vi "sensor_messung.vi"(8 "error in (no error)":errorcluster, 10 "Sensorkoord [P1 P2]":dbl[][](array[numeric]), 11 "Kreisquadrant in":refnum<class "Kreisquadrant.lvclass">) -> (0 "error out":errorcluster, 1 "Sensor auf Linie":bool, 2 "Schnittpunkt":dbl[](array[numeric]), 3 "Kreisquadrant out":refnum<class "Kreisquadrant.lvclass">)   [LabVIEW 2019, in "Kreisquadrant.lvclass"]
uses:
  Kreisquadrant.lvclass
  Kreisquadrant.lvclass/Kreisquadrant.ctl
  <vilib>/Analysis/baseanly.llb/Real Dot Product.vi
  <vilib>/Analysis/NI_AALPro.lvlib
  <vilib>/Analysis/NI_AALBase.lvlib
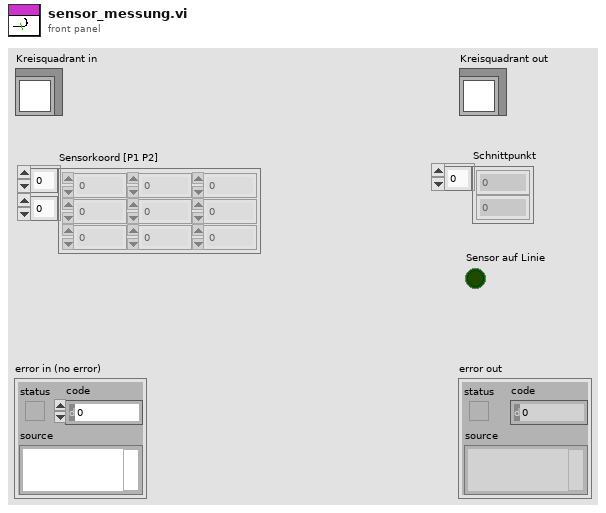
[diagram p1: front panel]
types:
  T1 = typedef "Quadrant.ctl" = enum16{"oben_rechts", "oben_links", "unten_links", "unten_rechts"}
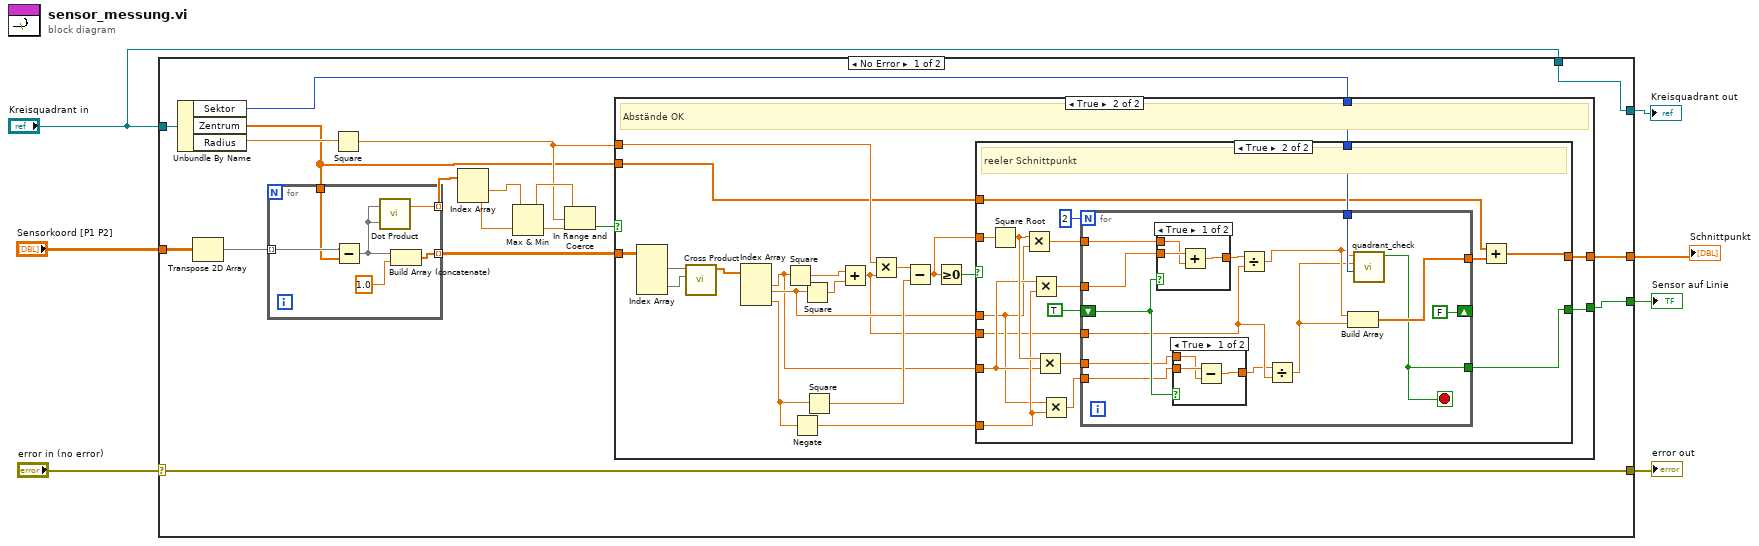
[diagram p0: block diagram]
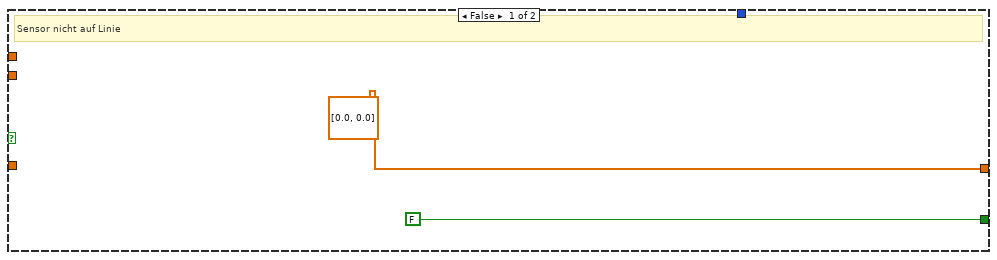
[diagram p2: hidden frame]
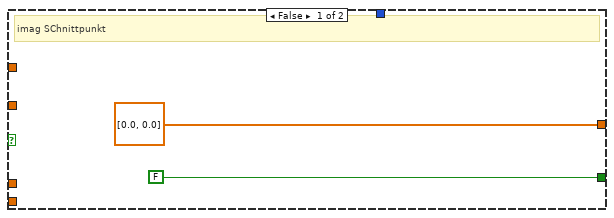
[diagram p3: hidden frame]
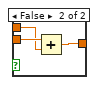
[diagram p4: hidden frame]
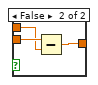
[diagram p5: hidden frame]
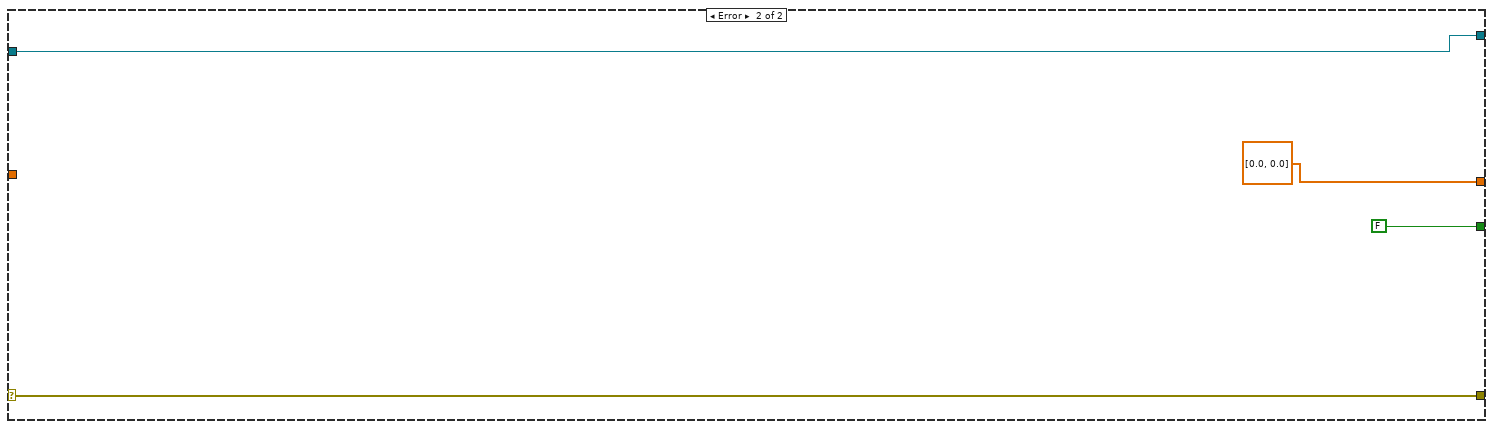
[diagram p6: hidden frame]
diagram:
  n1 = case shown="No Error" "error in (no error)" {
    selector: "error in (no error)" -> [w25 w102]
    tunnel: [w25 w102] -> w6
    tunnel: "Kreisquadrant in" -> [w24 w99]
    tunnel: "Sensorkoord [P1 P2]" -> [w23 _]
    tunnel: [w12 dbl[] [0.0, 0.0]] -> w4
    tunnel: [w13 FALSE ("Quadrant OK")] -> w3
    tunnel: [w9 w99] -> w2
    tunnel: "Kreisquadrant in" -> [w9 _]
    frame No Error {
      n2 = Unbundle By Name(w24) -> ("Sektor"=w10:T1, "Zentrum"=w8:dbl[], "Radius"=w20:dbl)
      n3 = Transpose 2D Array(2D array=w23) -> (transposed array=w22:dbl[][])
      n4 = for {
        tunnel: w22 -> [w98] mode=indexing
        tunnel: w8 -> [w97]
        tunnel: [w96] -> w21 mode=indexing
        tunnel: [w93] -> w19 mode=indexing
        n5 = Subtract(x=w98, y=w97) -> (x-y=w94:dbl[])
        n6 = call-poly <vilib>:"Dot Product.vi"("Y Vector"=w94, "X Vector"=w94) -> ("X * Y"=w93:dbl)  [unwired: 1 out]
        n7 = Build Array (concatenate)(w94, 1.0) -> (w96:dbl[])
      }
      n8 = Square(x=w20) -> (x^2=w11:dbl)
      n9 = Index Array(array=w19) -> (element #1=w18:dbl, element #2=w17:dbl)  [unwired: 2 in]
      n10 = Max & Min(x=w18, y=w17) -> (max(x,y)=w16:dbl, min(x,y)=w15:dbl)
      n11 = In Range and Coerce(upper limit=w16, x=w11, lower limit=w15) -> (In Range?=w14:bool)  [unwired: 1 out]
      n12 = case shown="True" w14 {
        tunnel: w21 -> [_ w47]
        tunnel: [FALSE w36] -> w13
        tunnel: [dbl[] [0.0, 0.0] w37] -> w12
        tunnel: w11 -> [_ w41]
        tunnel: w10 -> [_ w30]
        tunnel: w8 -> [_ w29]
        frame False {
          # "Sensor nicht auf Linie"
        }
        frame True {
          # "Abstände OK"
          n13 = Index Array(array=w47) -> (element #1=w46:dbl[], element #2=w45:dbl[])  [unwired: 4 in]
          n14 = call <vilib>:"Cross Product.vi"("B Vector"=w45, "A Vector"=w46) -> ("Cross Product"=w44:dbl[])  [unwired: 8 in, 1 out]
          n15 = Index Array(array=w44) -> (element #1=w33:dbl, element #2=w34:dbl, element #3=w32:dbl)  [unwired: 3 in]
          n16 = Square(x=w33) -> (x^2=w42:dbl)
          n17 = Negate(x=w32) -> (-x=w28:dbl)
          n18 = Square(x=w34) -> (x^2=w43:dbl)
          n19 = Square(x=w32) -> (x^2=w39:dbl)
          n20 = Add(x=w42, y=w43) -> (x+y=w31:dbl)
          n21 = Multiply(x=w41, y=w31) -> (x*y=w40:dbl)
          n22 = Subtract(x=w40, y=w39) -> (x-y=w35:dbl)
          n23 = Greater Or Equal To 0?(x=w35) -> (x >= 0?=w38:bool)
          n24 = case shown="True" w38 {
            tunnel: [dbl[] [0.0, 0.0] w50] -> w37
            tunnel: [FALSE w52] -> w36
            tunnel: w35 -> [_ w66]
            tunnel: w34 -> [_ w62]
            tunnel: w33 -> [_ w63]
            tunnel: w28 -> [_ w64]
            tunnel: w31 -> [_ w57]
            tunnel: w30 -> [_ w54]
            tunnel: w29 -> [_ w51]
            frame False {
              # "imag SChnittpunkt"
            }
            frame True {
              # "reeler Schnittpunkt"
              n25 = Square Root(x=w66) -> (sqrt(x)=w65:dbl)
              n26 = Multiply(x=w65, y=w62) -> (x*y=w58:dbl)
              n27 = Multiply(x=w63, y=w64) -> (x*y=w59:dbl)
              n28 = Multiply(x=w65, y=w63) -> (x*y=w55:dbl)
              n29 = Multiply(x=w62, y=w64) -> (x*y=w56:dbl)
              n30 = for {
                N: 2 -> [_]
                shift-right: [FALSE] -> _
                shift-left: TRUE -> [w76]
                tunnel: w59 -> [w80]
                tunnel: w58 -> [w79]
                tunnel: w57 -> [w73]
                tunnel: w56 -> [w75]
                tunnel: w55 -> [w74]
                tunnel: w54 -> [w71]
                tunnel: [w68] -> w53
                tunnel: [w67] -> w52
                stop <- w67 stop-if-true
                n31 = case shown="True" w76 {
                  tunnel: w80 -> [w89 w92]
                  tunnel: w79 -> [w88 w91]
                  tunnel: [w87 w90] -> w78
                  frame True {
                    n32 = Add(x=w89, y=w88) -> (x+y=w87:dbl)
                  }
                  frame False {
                    n33 = Subtract(x=w92, y=w91) -> (x-y=w90:dbl)
                  }
                }
                n34 = case shown="True" w76 {
                  tunnel: w75 -> [w83 w86]
                  tunnel: w74 -> [w82 w85]
                  tunnel: [w81 w84] -> w72
                  frame True {
                    n35 = Subtract(x=w83, y=w82) -> (x-y=w81:dbl)
                  }
                  frame False {
                    n36 = Add(x=w86, y=w85) -> (x+y=w84:dbl)
                  }
                }
                n37 = Divide(x=w78, y=w73) -> (x/y=w70:dbl)
                n38 = Divide(x=w72, y=w73) -> (x/y=w69:dbl)
                n39 = Build Array(w70, w69) -> (w68:dbl[])
                n40 = call "quadrant_check.vi"("Sektor"=w71, "y"=w69, "x"=w70) -> ("Quadrant OK"=w67:bool)  [unwired: 8 in]
              }
              n41 = Add(x=w51, y=w53) -> (x+y=w50:dbl[])
            }
          }
        }
      }
    }
    frame Error {
    }
  }
  "error out" <- w6
  "Kreisquadrant out" <- w2
  "Sensor auf Linie" <- w3
  "Schnittpunkt" <- w4
